vi "LinearQuadraticRegulator_Reset.vi"(11 "in LinearQuadraticRegulator":T1) -> (3 "out LinearQuadraticRegulator":T1)   [LabVIEW 2019, in "Trajectory_Library.lvlib"]
doc: "Resets the controller.\n\nInputs:\n -- LinearQuadraticRegulator -- controller data cluster\n\nOutputs:\n -- outLinearQuadraticRegulator -- updated controller data cluster"
uses:
  Trajectory_Library.lvlib
  LINEAR_QUADRATIC_REGULATOR.ctl
  <vilib>/Analysis/Matrix/Datatypes/RealMatrix.ctl
  <vilib>/Analysis/Matrix/NI_Matrix.lvlib
panel:
  # "Ref State <States,1>"
  # "Comp and capped \noutput <Inputs,1>"
  # "Controller gain\n<Inputs,States>"
  # "Ref State <States,1>"
  # "Comp and capped \noutput <Inputs,1>"
  # "Controller gain\n<Inputs,States>"
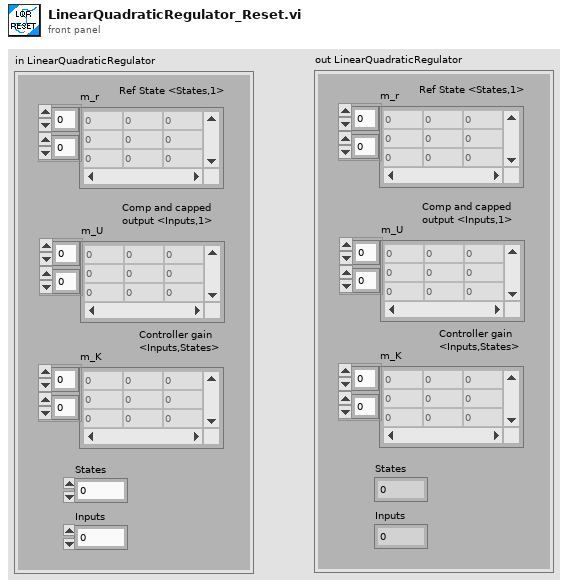
[diagram p1: front panel]
types:
  T1 = typedef "Trajectory_Library.lvlib/LINEAR_QUADRATIC_REGULATOR.ctl" = cluster{"m_r":T2, "m_U":T2, "m_K":T2, "States":i32, "Inputs":i32}
  T2 = typedef "NI_Matrix.lvlib/RealMatrix.ctl" = dbl[][]
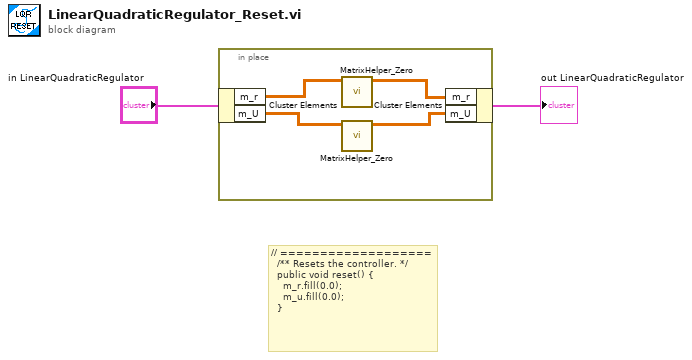
[diagram p0: block diagram]
diagram:
  # "// ===================\n  /** Resets the controller. */\n  public void reset() {\n    m_r.fill(0.0);\n    m_u.fill(0.0);\n  }"
  n1 = in-place {
    n2 = in-place-cluster #1("in LinearQuadraticRegulator") -> ("m_r"=w6:T2, "m_U"=w5:T2)
    n3 = call "MatrixHelper_Zero.vi"("input matrix"=w6) -> ("output matrix"=w4:T2)  [unwired: 10 in]
    n4 = call "MatrixHelper_Zero.vi"("input matrix"=w5) -> ("output matrix"=w3:T2)  [unwired: 10 in]
    n5 = in-place-cluster #1("m_r"=w4, "m_U"=w3) -> (→"out LinearQuadraticRegulator":T1)
  }
